vi "Intan_StreamData_parallelLoop.vi"(0 "VISA resource name":refnum<visa-resource-name>, 1 "refnum in":refnum<file>, 3 "stop":bool, 4 "Save Binary Data":bool, 5 "error in":errorcluster, 7 "byte order":T4(ring)=enum."little-endian", 8 "hdr fpath":path, 11 "DT_scale (sec)":dbl=0.01, 12 "aux file ref num":refnum<file>, 14 "save aux file":bool) -> (6 "N data scans to read (VISA)":i32=20, 10 "Nbytes VISA read":u32, 13 "VISA read iter":i32, 19 "error out":errorcluster)   [LabVIEW 2015]
doc: "Stream data to disk and user friendly display. Data is scaled and filtered prior to display.\n\nThis VI uses parallel while loop architecture: 1 loop reads from serial stream and saves raw bytes to disk; the other loop processes the data in chunk, scaling and filtering, then displays."
uses:
  zip_swcircularbuffer1_0_19b/Circular Buffer/Controls/Circular Buffer Status.ctl
  zip_swcircularbuffer1_0_19b/Circular Buffer/Controls/Circular Buffer Operations.ctl
  <vilib>/Utility/error.llb/DialogType.ctl
  zip_swcircularbuffer1_0_19b/Circular Buffer/Instance VIs/Circular Buffer(1D U16).vi
  zip_swcircularbuffer1_0_19b/Circular Buffer/Circular Buffer.lvlib
panel:
  out "setscaleresult":dbl
  out "UpdateCode":i16
  out "xmax_init":dbl
  out "offset_init":dbl
  out "increment_init":dbl
  out "xmin_init":dbl
  out "NchansChanged":bool
  out "DispLengthChanged":bool
  out "XscaleRollover":bool
  in  "Buffer Read Interval (ms)":dbl=100.0
  out "Picture":picture
  in  "Display Update interval (ms)":dbl=100.0
  in  "ChartDisplayLength (s)":dbl=5.0
  out "FS (Hz)":dbl
  out "YtxtLabelsAll":string[](array[string])
  out "error code out":i32 format="%0.0f"
  out "StopLoopsMaster":bool
  in  "Channel Select":bool
  in  "Display Chans":i32[](listbox)=[1, 4, 13, 14, 15, 16, 17, 22]
  in  "Center Traces":bool
  out "non integer read":bool
  out "N_u16s  write to buf":i32
  out "Nelements to read from buf":dbl
  out "display iter":i32
  out "% buffer full":dbl(slide) scale=0.0..100.0
  in  "Ring Buffer Size":T1={"Samples per Channel"=640000, "Channels"=0}
  out "buffer underflow":bool
  out "Buffer Status  (read)":T2
  out "buffer overflow":bool
  out "Buffer Status (write)":T2
  out "Save status":bool
  in  "Filter settings":T3={"LP Filter On/Off"=TRUE, "LP Cutoff (Hz)"=40.0, "HP Filter On/Off"=TRUE, "HP Cutoff (Hz)"=0.5, "Bandstop On/Off"=TRUE, "fl Cutoff (Hz)"=48.0, "fh Cutoff (Hz) "=52.0}
  out "N data scans to display":u16=20
  in  "offset factor":dbl=1.0
  in  "DisplayScale (uV/div)":u16(ring)=1 items=["6400", "3200", "1600", "800", "400", "200", "100", "50", "25"]
  in  "bytes per scan":i32=72
  out "timestamp_array":i32[](array[numeric])
  out "aux_cmd_array":i32[][](array[numeric])
  out "binary data (from VISA read)":u16[](array[numeric])
  in  "Nchans":i32=32
  in  "start stream (Teensy char)":string="s"
  in  "pause stream (Teensy char)":string="p"
  out "Intan Streaming Data":dbl[][](graph)
  out "Text response":string
  # "Intan-Teensy Bioelectric Module: Data Stream and Visualization"
  # "1-D data stream \nreformatted  to 2-D"
  # "Display Settings"
  # "xscale controls"
  # "Free Select"
  # "Show All"
  # "Ring Buffer Status"
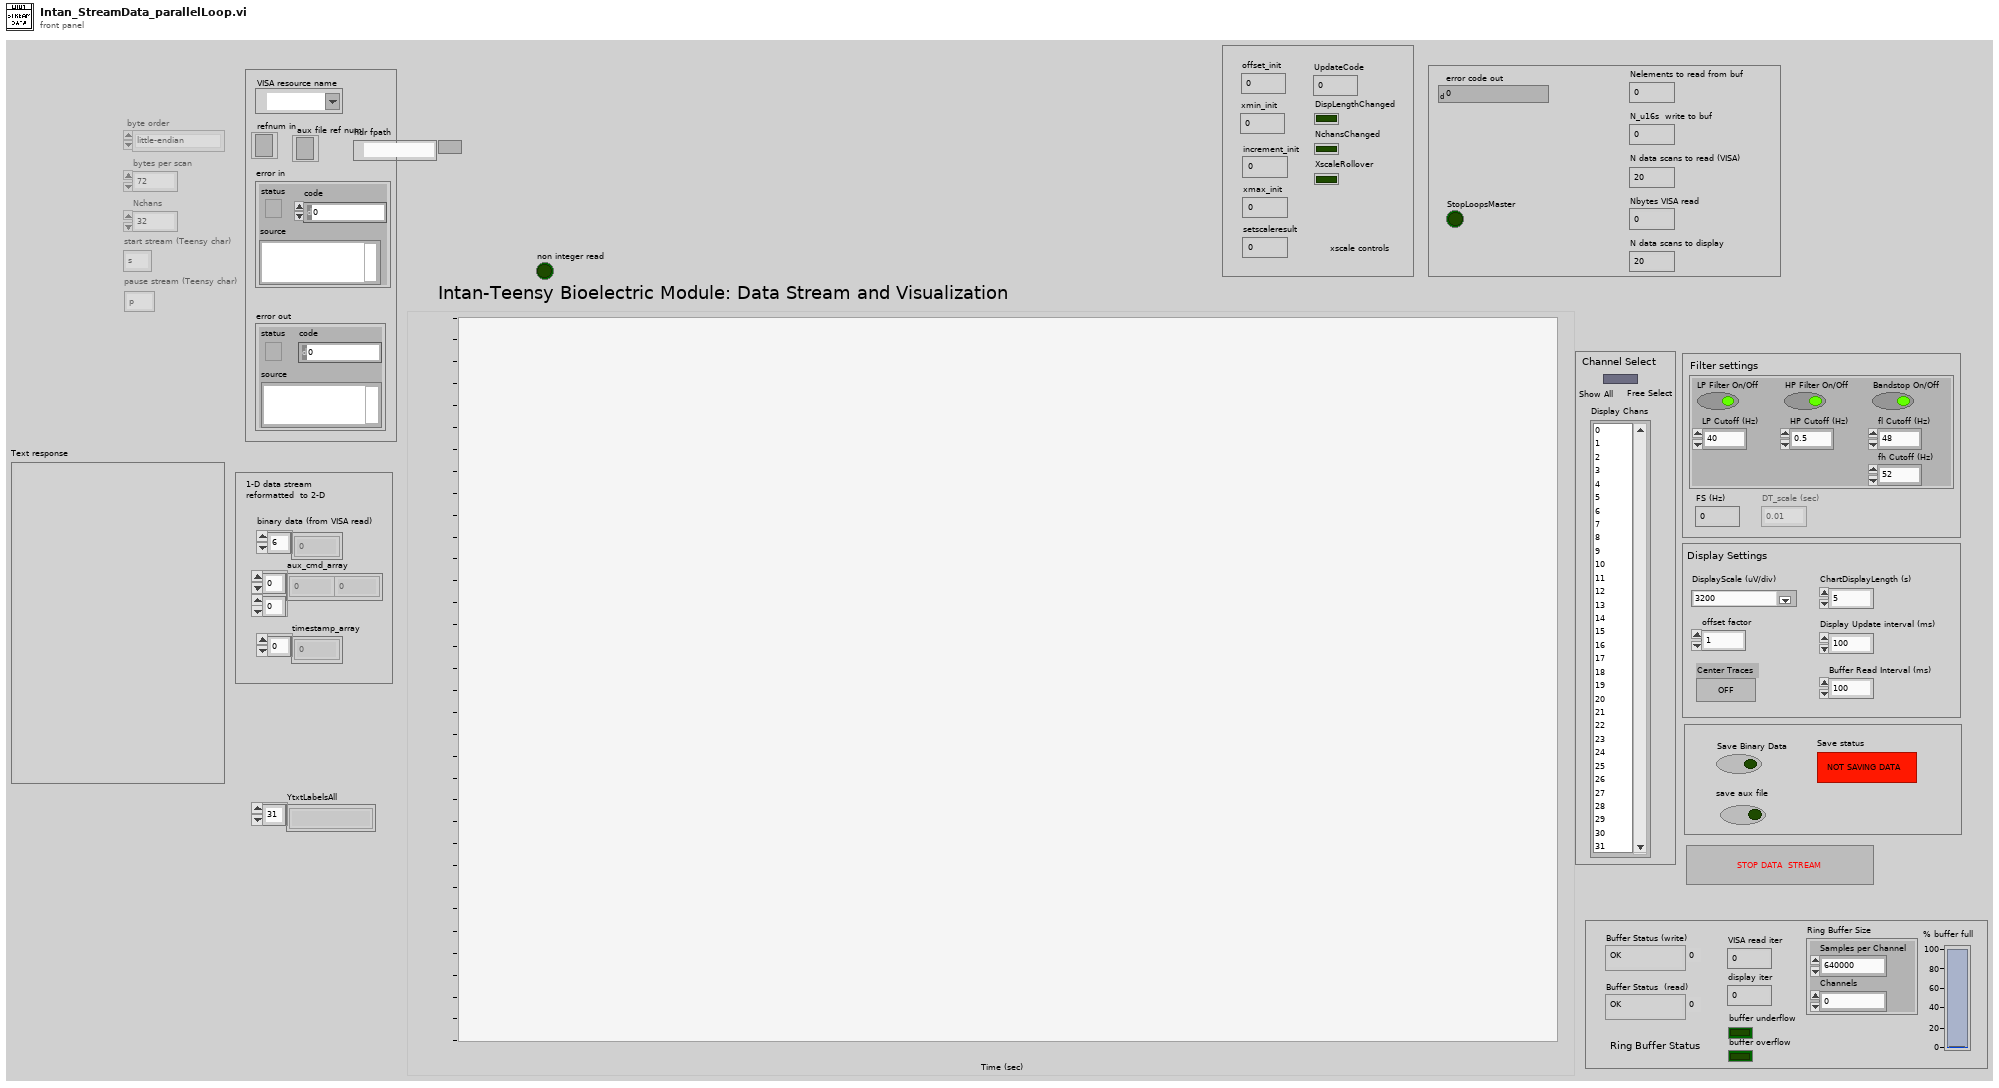
[diagram p1: front panel]
types:
  T1 = cluster{"Samples per Channel":u32, "Channels":u32}
  T2 = typedef "Circular Buffer.lvlib/Circular Buffer Status.ctl" = enum16{"OK", "Overflow", "Underflow"}
  T3 = cluster{"LP Filter On/Off":bool, "LP Cutoff (Hz)":dbl, "HP Filter On/Off":bool, "HP Cutoff (Hz)":dbl, "Bandstop On/Off":bool, "fl Cutoff (Hz)":dbl, "fh Cutoff (Hz) ":dbl}
  T4 = enum16{"big-endian, network order", "native, host order", "little-endian"}
  T5 = typedef "Circular Buffer.lvlib/Circular Buffer Operations.ctl" = enum16{"Initialize", "Get Backlog", "Write", "Read (continuous)", "Read (most recent)"}
  T6 = typedef "LVRectTypeDef.ctl" = cluster{"Left":i16, "Top":i16, "Right":i16, "Bottom":i16}
  T7 = typedef "DialogType.ctl" = u16
  T8 = cluster{"XScale.Minimum":dbl, "XScale.Maximum":dbl, "XScale.Increment":dbl, "Nchannels":i32}
  T9 = cluster{"Maximum":dbl, dbl, dbl, dbl, dbl, dbl, "YscleMark":dbl, "Increment":dbl}
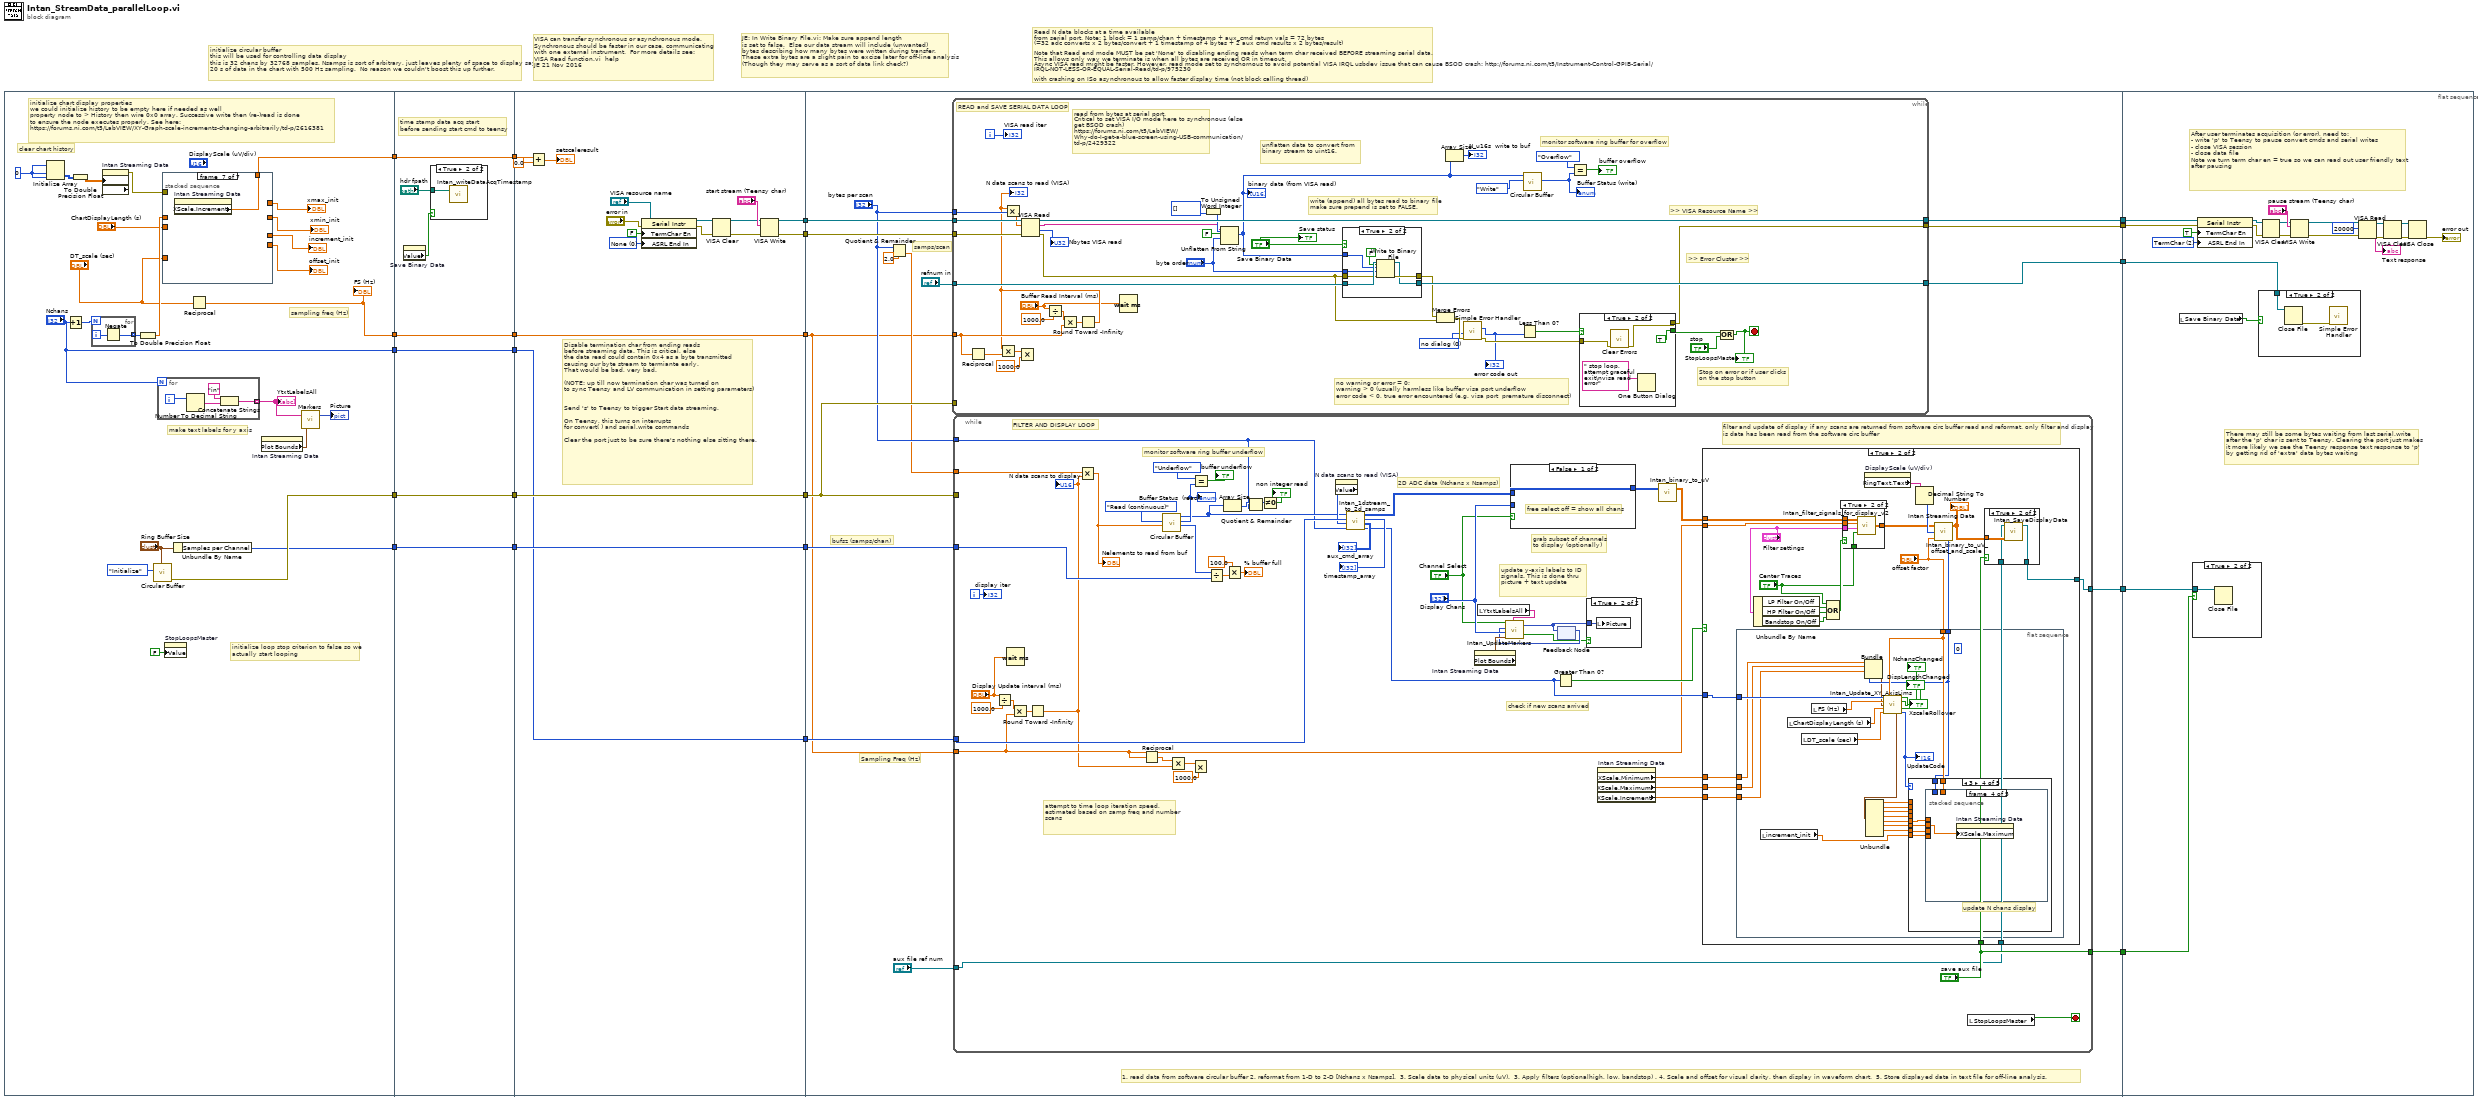
[diagram p0: block diagram]
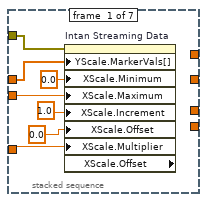
[diagram p2: hidden frame]
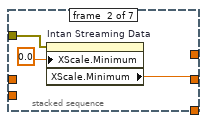
[diagram p3: hidden frame]
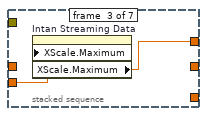
[diagram p4: hidden frame]
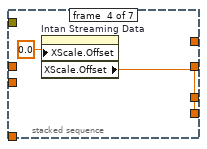
[diagram p5: hidden frame]
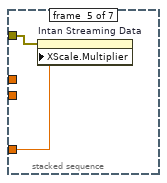
[diagram p6: hidden frame]
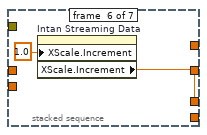
[diagram p7: hidden frame]
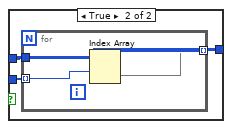
[diagram p10: hidden frame]
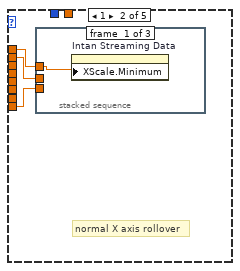
[diagram p13: hidden frame]
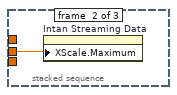
[diagram p14: hidden frame]
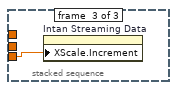
[diagram p15: hidden frame]
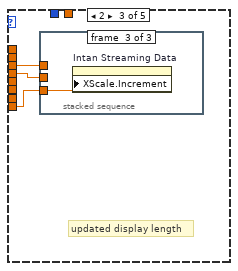
[diagram p16: hidden frame]
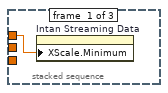
[diagram p17: hidden frame]
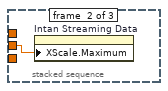
[diagram p18: hidden frame]
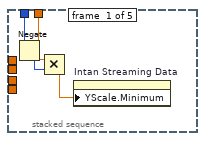
[diagram p19: hidden frame]
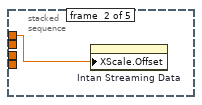
[diagram p20: hidden frame]
diagram:
  # "Read N data blocks at a time available\nfrom serial port. Note: 1 block = 1 samp/chan + timestamp + aux_cmd return vals = 72 bytes \n(=32 adc converts x 2 bytes/convert + 1 timestamp of 4 bytes + 2 aux cmd results x 2 bytes/result) \n\nNote that Read end mode MUST be set 'None' to disabling ending reads when term char received BEFORE streaming serial data.  \nThis allows only way we terminate is when all bytes are received OR in timeout.  \nAsync VISA read might be faster. However, read mode set to synchornous to avoid potential VISA IRQL usbdev issue that can cause BSOD crash: http://forums.ni.com/t5/Instrument-Control-GPIB-Serial/IRQL-NOT-LESS-OR-EQUAL-Serial-Read/td-p/975230\n\nwith crashing on ISo asynchronous to allow faster display time (not block calling thread)"
  # "initialize circular buffer\nthis will be used for controlling data display\nthis is 32 chans by 32768 samples. Nsamps is sort of arbitrary, just leaves plenty of space to display say\n20 s of data in the chart with 500 Hz sampling.  No reason we couldn't boost this up further."
  # "JE: In Write Binary File.vi: Make sure append length \nis set to false.  Else our data stream will include (unwanted)\nbytes describing how many bytes were written during transfer.\nThese extra bytes are a slight pain to excise later for off-line analysis\n(Though they may serve as a sort of data link check?)"
  # "VISA can transfer synchronous or asynchronous mode.\nSynchronous should be faster in our case, communicating\nwith one external instrument.  For more details see: \nVISA Read function.vi  help \nJE 21 Nov 2016"
  n1 = flat-sequence {
    tunnel: [w42] -> w10
    tunnel: [w40] -> w8
    tunnel: ["Nchans"] -> w6
    tunnel: [w34] -> w4
    tunnel: [w22] -> w2
    tunnel: w10 -> [w77]
    tunnel: [w77] -> w9
    tunnel: w8 -> [w76]
    tunnel: [w76] -> w7
    tunnel: w6 -> [w75]
    tunnel: [w75] -> w5
    tunnel: w4 -> [w74]
    tunnel: [w74] -> w3
    tunnel: w2 -> [w73]
    tunnel: [w73] -> w1
    tunnel: [w86] -> w19
    tunnel: [w87] -> w18
    tunnel: [w85] -> w17
    tunnel: w9 -> [w85]
    tunnel: [w84] -> w16
    tunnel: w7 -> [w84]
    tunnel: w5 -> [w83]
    tunnel: [w83] -> w15
    tunnel: [w82] -> w14
    tunnel: w3 -> [w82]
    tunnel: w1 -> [w81]
    tunnel: [w108] -> w21
    tunnel: [w111] -> w20
    tunnel: w19 -> [w109]
    tunnel: w18 -> [w110]
    tunnel: w17 -> [w107]
    tunnel: w16 -> [w105]
    tunnel: w15 -> [w104]
    tunnel: w14 -> [w101]
    tunnel: [w100] -> w13
    tunnel: [w98] -> w12
    tunnel: [w97] -> w11
    tunnel: w21 -> [w331]
    tunnel: w20 -> [w344]
    tunnel: w13 -> [w326]
    tunnel: w12 -> [w325]
    tunnel: w11 -> [w324]
    frame #0 {
      w33 = 0 ("Dimension Size")
      # "clear chart history"
      # "initialize loop stop criterion to false so we\nactually start looping"
      # "make text labels for y axis"
      # "sampling freq (Hz)"
      # "initialize chart display properties\nwe could initialize history to be empty here if needed as well\nproperty node to > History then wire 0x0 array. Successive write then (re-)read is done\nto ensure the node executes properly. See here:\nhttps://forums.ni.com/t5/LabVIEW/XY-Graph-scale-increments-changing-arbitrarily/td-p/2616381"
      n2 = Initialize Array(w33, w33, w33) -> (w32:i32[][])
      n3 = Increment(x="Nchans") -> (x+1=w44:i32)
      n4 = To Double Precision Float(number=w32) -> (double precision float=w30:dbl[][])
      n5 = for {
        N: w44 -> [_]
        tunnel: [w69] -> w45 mode=indexing
        i -> [w70]
        n6 = Negate(x=w70) -> (-x=w69:i32)
      }
      n7 = property on="Intan Streaming Data" class="WFChart (strict)" props=["History Data", "History Data"]("History Data"=w30) -> (error out=w29:errorcluster)  [unwired: 2 in, 2 out]
      n8 = To Double Precision Float(number=w45) -> (double precision float=w31:dbl[])
      n9 = call-poly "Circular Buffer.vi"("Buffer Size"="Ring Buffer Size", "Operation"=Circular_Buffer_Operations."Initialize") -> ("error out"=w42:errorcluster)  [unwired: 6 in, 3 out]
      n10 = for {
        N: "Nchans" -> [_]
        tunnel: [w66] -> w37 mode=indexing
        i -> [w65]
        n11 = Number To Decimal String(number=w65) -> (decimal integer string=w68:string)  [unwired: 1 in]
        n12 = Concatenate Strings("in" ("string"), w68) -> (w66:string)
      }
      "YtxtLabelsAll" <- w37
      n13 = stacked-sequence {
        tunnel: w31 -> [w52 _ _ _ _ _ _]
        tunnel: w29 -> [w51 w54 _ _ w60 _ _]
        tunnel: "ChartDisplayLength (s)" -> [w49 _ w57 _ _ _ _]
        tunnel: "DT_scale (sec)" -> [w48 _ _ _ w61 _ _]
        tunnel: [_ _ w56 _ _ _ _] -> w23
        tunnel: [_ w55 _ _ _ _ _] -> w26
        tunnel: [_ _ _ _ _ w62 _] -> w25
        tunnel: [_ _ _ w58 _ _ _] -> w24
        tunnel: [_ _ _ _ _ _ w64] -> w22
        frame #0 {
          n14 = property on="Intan Streaming Data" class="WFChart (strict)" props=["YScale", "MarkerVals[]", "XScale", "Minimum", "XScale", "Maximum", "XScale", "Increment", "XScale", "Offset", "XScale", "Multiplier", "XScale", "Offset"](error in=w51, "YScale.MarkerVals[]"=w52, "XScale.Minimum"=0.0 ("X Scale.Range:Minimum"), "XScale.Maximum"=w49, "XScale.Increment"=1.0 ("X Scale.Range:Minimum"), "XScale.Offset"=0.0 ("X Scale.Range:Minimum"), "XScale.Multiplier"=w48) -> ()  [unwired: 1 in, 3 out]
        }
        frame #1 {
          n15 = property on="Intan Streaming Data" class="WFChart (strict)"(error in=w54, "XScale.Minimum"=0.0 ("X Scale.Range:Minimum")) -> ("XScale.Minimum"=w55:dbl)  [unwired: 1 in, 2 out]
        }
        frame #2 {
          n16 = property on="Intan Streaming Data" class="WFChart (strict)"("XScale.Maximum"=w57) -> ("XScale.Maximum"=w56:dbl)  [unwired: 2 in, 2 out]
        }
        frame #3 {
          n17 = property on="Intan Streaming Data" class="WFChart (strict)"("XScale.Offset"=0.0 ("X Scale.Offset and Multiplier:Offset")) -> ("XScale.Offset"=w58:dbl)  [unwired: 2 in, 2 out]
        }
        frame #4 {
          n18 = property on="Intan Streaming Data" class="WFChart (strict)"(error in=w60, "XScale.Multiplier"=w61) -> ()  [unwired: 1 in, 2 out]
        }
        frame #5 {
          n19 = property on="Intan Streaming Data" class="WFChart (strict)"("XScale.Increment"=1.0 ("X Scale.Range:Increment")) -> ("XScale.Increment"=w62:dbl)  [unwired: 2 in, 2 out]
        }
        frame #6 {
          n20 = property on="Intan Streaming Data" class="WFChart (strict)"() -> ("XScale.Increment"=w64:dbl)  [unwired: 2 in, 2 out]
        }
      }
      "xmin_init" <- w26
      "increment_init" <- w25
      "offset_init" <- w24
      "xmax_init" <- w23
      n21 = property on="StopLoopsMaster" class="Bool (strict)"("Value"=FALSE ("StopLoopsMaster")) -> ()  [unwired: 2 in, 2 out]
      n22 = Unbundle By Name("Ring Buffer Size") -> ("Samples per Channel"=w40:u32)
      n23 = Reciprocal(x="DT_scale (sec)") -> (1/x=w34:dbl)
      "FS (Hz)" <- w34
      n24 = property on="Intan Streaming Data" class="WFChart (strict)"() -> ("Plot Bounds"=w35:T6)  [unwired: 2 in, 2 out]
      n25 = call "Markers.vi"("plot bounds"=w35, "Array"=w37) -> ("Picture"=→"Picture":picture)  [unwired: 1 out]
    }
    frame #1 {
      # "time stamp data acq start\nbefore sending start cmd to teensy"
      n26 = property on="Save Binary Data" class="Bool (strict)"() -> ("Value"=w72:bool)  [unwired: 2 in, 2 out]
      n27 = case shown="True" w72 {
        tunnel: "hdr fpath" -> [_ w78]
        frame False {
        }
        frame True {
          n28 = call "Intan_writeDataAcqTimestamp.vi"("hdr fpath"=w78) -> ()  [unwired: 2 in, 1 out]
        }
      }
    }
    frame #2 {
      w92 = u16 0 items=["None", "Last Bit", "TermChar"] ("Serial Settings:End Mode for Reads")
      # "Disable termination char from ending reads\nbefore streaming data. This is critical, else\nthe data read could contain 0x4 as a byte transmitted\ncausing our byte stream to termiante early.\nThat would be bad, very bad.\n\n(NOTE: up till now termination char was turned on\nto sync Teensy and LV communication in setting parameters)\n\n\nSend 's' to Teensy to trigger Start data streaming.  \n\nOn Teensy, this turns on interrupts\nfor convert( ) and serial.write commands\n\nClear the port just to be sure there's nothing else sitting there."
      n29 = Add(x=w81, y=0.0) -> (x+y=→"setscaleresult":dbl)
      n30 = property class="Serial Instr"(reference="VISA resource name", error in="error in", "TermChar En"=FALSE ("Message Based Settings:Termination Character Enable"), "ASRL End In"=w92) -> (reference out=w91:refnum<visa-resource-name>, error out=w90:errorcluster)
      n31 = VISA Clear(VISA resource name=w91, error in (no error)=w90) -> (VISA resource name out=w89:refnum<visa-resource-name>, error out=w88:errorcluster)
      n32 = VISA Write(VISA resource name=w89, write buffer="start stream (Teensy char)", error in (no error)=w88) -> (VISA resource name out=w87:refnum<visa-resource-name>, error out=w86:errorcluster)  [unwired: 1 out]
    }
    frame #3 {
      # "1. read data from software circular buffer 2. reformat from 1-D to 2-D [Nchans x Nsamps].  3. Scale data to physical units (uV).  3. Apply filters (optionalhigh, low, bandstop) . 4. Scale and offset for visual clarity, then display in waveform chart.  5. Store displayed data in text file for off-line analysis."
      # "Sampling Freq (Hz)"
      # "bufsz (samps/chan)"
      # "samps/scan"
      n33 = Quotient & Remainder(x="bytes per scan", y=2.0) -> (floor(x/y)=w102:dbl)  [unwired: 1 out]
      n34 = while {
        tunnel: [w307] -> w108
        tunnel: [w305] -> w111
        tunnel: w109 -> [w301]
        tunnel: "refnum in" -> [w304]
        tunnel: w110 -> [w302]
        tunnel: w107 -> [_]
        tunnel: "bytes per scan" -> [w286]
        tunnel: w101 -> [w269]
        tunnel: [w273] -> w98
        i -> [w303]
        stop <- w306 stop-if-true
        w279 = T7 0 items=["no dialog", "OK message", "continue or stop message", "OK message + warnings", "continue/stop + warnings"] ("type of dialog (OK msg:1)")
        # "no warning or error = 0;\nwarning > 0 (usually harmless like buffer visa port underflow\nerror code < 0, true error encountered (e.g. visa port  premature disconnect)"
        # "READ and SAVE SERIAL DATA LOOP"
        # "monitor software ring buffer for overflow"
        # "write (append) all bytes read to binary file\nmake sure prepend is set to FALSE."
        # "unflatten data to convert from binary stream to uint16."
        # "Stop on error or if user clicks \non the stop button"
        # ">> Error Cluster >>"
        # ">> VISA Resource Name >>"
        # "read from bytes at serial port.\nCritical to set VISA I/O mode here to synchronous (else get BSOD crash)\nhttps://forums.ni.com/t5/LabVIEW/Why-do-I-get-a-blue-screen-using-USB-communication/td-p/2429322"
        n35 = Reciprocal(x=w269) -> (1/x=w283:dbl)
        n36 = Divide(x="Buffer Read Interval (ms)", y=1000.0) -> (x/y=w271:dbl)
        n37 = Multiply(x=w271, y=w269) -> (x*y=w272:dbl)
        n38 = Round Toward -Infinity(1:w272) -> (0:w268:dbl)
        "N data scans to read (VISA)" <- w268
        n39 = Multiply(x=w268, y=w283) -> (x*y=w285:dbl)
        n40 = Multiply(x=w268, y=w286) -> (x*y=w287:dbl)
        n41 = Multiply(x=w285, y=1000.0) -> ()  [unwired: 1 out]
        n42 = VISA Read(VISA resource name=w302, byte count=w287, error in (no error)=w301) -> (VISA resource name out=w307:refnum<visa-resource-name>, read buffer=w295:string, return count=→"Nbytes VISA read":u32, error out=w281:errorcluster)
        n43 = Wait (ms)(milliseconds to wait="Buffer Read Interval (ms)") -> ()  [unwired: 1 out]
        n44 = To Unsigned Word Integer(number=i16[] []) -> (unsigned 16bit integer=w297:u16[])
        n45 = Unflatten From String(type=w297, binary string=w295, data includes array or string size? (T)=FALSE, byte order (0:big-endian, network order)="byte order") -> (value=w289:u16[])  [unwired: 1 in, 2 out]
        "binary data (from VISA read)" <- w289
        n46 = case shown="True" "Save Binary Data" {
          tunnel: [w315 w322] -> w282
          tunnel: [w314 w321] -> w305
          tunnel: w304 -> [w314 w320]
          tunnel: w281 -> [w315 w319]
          tunnel: "byte order" -> [_ w317]
          tunnel: w289 -> [_ w316]
          frame False {
          }
          frame True {
            n47 = Write to Binary File(file (use dialog)=w320, data=w316, error in=w319, 5:FALSE ("prepend array or string size? (T)"), 9:w317) -> (refnum out=w321:refnum<file>, error out=w322:errorcluster)  [unwired: 1 in, 1 out]
          }
        }
        n48 = Merge Errors(w282, w281) -> (w280:errorcluster)
        n49 = Array Size(array=w289) -> (size(s)=→"N_u16s  write to buf":i32)
        n50 = call <vilib>:"Simple Error Handler.vi"("type of dialog (OK msg:1)"=w279, "error in (no error)"=w280) -> ("code out"=w276:i32, "error out"=w277:errorcluster)  [unwired: 3 in, 3 out]
        "error code out" <- w276
        n51 = Less Than 0?(x=w276) -> (x < 0?=w274:bool)
        n52 = call-poly "Circular Buffer.vi"("Operation"=Circular_Buffer_Operations."Write", "Data In"=w289) -> ("Buffer Status"=w291:T2)  [unwired: 6 in, 3 out]
        "Buffer Status (write)" <- w291
        n53 = Equal?(x=Circular_Buffer_Status."Overflow" ("y"), y=w291) -> (x = y?=→"buffer overflow":bool)
        n54 = case shown="True" w274 {
          tunnel: w277 -> [w308 w312]
          tunnel: [FALSE TRUE] -> w275
          tunnel: [w308 w310] -> w273
          frame False {
          }
          frame True {
            n55 = call <vilib>:"Clear Errors.vi"("error in (no error)"=w312) -> ("error out"=w310:errorcluster)  [unwired: 5 in, 1 out]
            n56 = One Button Dialog(message=" stop loop, attempt graceful exit\nvisa read error") -> ()  [unwired: 1 in, 1 out]
          }
        }
        n57 = Compound Arithmetic op=OR(w275, "stop") -> (w306:bool)
        "StopLoopsMaster" <- w306
        "VISA read iter" <- w303
        "Save status" <- "Save Binary Data"
      }
      n58 = while {
        tunnel: w107 -> [_]
        tunnel: w105 -> [w156]
        tunnel: w104 -> [w152]
        tunnel: "bytes per scan" -> [w142]
        tunnel: w101 -> [w121]
        tunnel: w102 -> [w148]
        tunnel: [w127] -> w100
        tunnel: "aux file ref num" -> [w126]
        tunnel: ["save aux file"] -> w97
        i -> [w149]
        stop <- w124 stop-if-true
        # "2D ADC data (Nchans x Nsamps)"
        # "check if new scans arrived"
        # "grab subset of channels\nto display (optionally)"
        # "update y-axis labels to ID signals. This is done thru picture + text update"
        # "FILTER AND DISPLAY LOOP"
        # "attempt to time loop iteration speed,\nestimated based on samp freq and number scans"
        # "filter and update of display if any scans are returned from software circ buffer read and reformat. only filter and display is data has been read from the software circ buffer"
        # "monitor software ring buffer underflow"
        n59 = Divide(x="Display Update interval (ms)", y=1000.0) -> (x/y=w118:dbl)
        n60 = Wait (ms)(milliseconds to wait="Display Update interval (ms)") -> ()  [unwired: 1 out]
        n61 = Multiply(x=w118, y=w121) -> (x*y=w120:dbl)
        n62 = Round Toward -Infinity(1:w120) -> (0:w119:dbl)
        "N data scans to display" <- w119
        n63 = Multiply(x=w148, y=w119) -> (x*y=w147:dbl)
        "Nelements to read from buf" <- w147
        n64 = Reciprocal(x=w121) -> (1/x=w139:dbl)
        n65 = call-poly "Circular Buffer.vi"("Read Size"=w147, "Operation"=Circular_Buffer_Operations."Read (continuous)") -> ("Elements Remaining"=w157:i32, "Buffer Status"=w159:T2, "Data Out"=w144:u16[])  [unwired: 6 in, 1 out]
        "Buffer Status  (read)" <- w159
        n66 = Multiply(x=w139, y=w119) -> (x*y=w138:dbl)
        n67 = Multiply(x=w138, y=1000.0) -> ()  [unwired: 1 out]
        n68 = Equal?(x=Circular_Buffer_Status."Underflow" ("y"), y=w159) -> (x = y?=→"buffer underflow":bool)
        n69 = Divide(x=w157, y=w156) -> (x/y=w155:dbl)
        n70 = Array Size(array=w144) -> (size(s)=w143:i32)
        n71 = Multiply(x=100.0, y=w155) -> (x*y=→"% buffer full":dbl)
        n72 = Quotient & Remainder(x=w143, y=w142) -> (x-y*floor(x/y)=w141:i32)  [unwired: 1 out]
        n73 = Not Equal To 0?(x=w141) -> (x != 0?=→"non integer read":bool)
        n74 = property on="N data scans to read (VISA)" class="DigNum (strict)"() -> ("Value"=w146:i32)  [unwired: 2 in, 2 out]
        n75 = call "Intan_1dstream_to_2d_samps.vi"("bytes per scan"=w142, "N data scans to read"=w146, "Nchans"=w152, "1-D  data in"=w144) -> ("Nscans read"=w125:i32, "aux_cmd_array"=→"aux_cmd_array":i32[][], "timestamp_array"=→"timestamp_array":i32[], "2d ADCdata_array out"=w136:u16[][])  [unwired: 2 in, 2 out]
        n76 = property on="Intan Streaming Data" class="WFChart (strict)"() -> ("Plot Bounds"=w133:T6)  [unwired: 2 in, 2 out]
        n77 = local read "YtxtLabelsAll"() -> (w122:string[])
        n78 = case shown="False" "Channel Select" {
          tunnel: w136 -> [w163 w166]
          tunnel: [w163 w165] -> w123
          tunnel: "Display Chans" -> [_ w164]
          frame False {
            # "free select off = show all chans"
          }
          frame True {
            n79 = for {
              tunnel: w166 -> [w169]
              tunnel: w164 -> [w167] mode=indexing
              tunnel: [w168] -> w165 mode=indexing
              n80 = Index Array(array=w169, index (row)=w167) -> (element=w168:u16[])  [unwired: 1 in]
            }
          }
        }
        n81 = Greater Than 0?(x=w125) -> (x > 0?=w145:bool)
        n82 = feedback #1() -> (w132:picture)  [unwired: 1 in]
        n83 = call "Intan_UpdateMarkers.vi"("Free Select Chans"="Channel Select", "Picture In"=w132, "Display Chans"="Display Chans", "plot bounds"=w133, "YtxtLabelsAll"=w122) -> ("Picture Out"=w129:picture, "update labels"=w130:bool)
        n84 = feedback-in #1(w129) -> ()
        n85 = case shown="True" w130 {
          tunnel: w129 -> [_ w162]
          frame False {
          }
          frame True {
            n86 = local write "Picture"(w162) -> ()
          }
        }
        n87 = property on="Intan Streaming Data" class="WFChart (strict)"() -> ("XScale.Minimum"=w115:dbl, "XScale.Maximum"=w114:dbl, "XScale.Increment"=w113:dbl)  [unwired: 2 in, 2 out]
        n88 = call "Intan_binary_to_uV.vi"("2d ADC binary data"=w123) -> ("Scaled Data (uV)"=w135:dbl[][])  [unwired: 2 in]
        n89 = case shown="True" w145 {
          tunnel: w121 -> [_ w190]
          tunnel: w135 -> [_ w188]
          tunnel: [w170 w181] -> w127
          tunnel: "save aux file" -> [_ w180]
          tunnel: w126 -> [w170 w179]
          tunnel: w125 -> [_ w177]
          tunnel: w115 -> [_ w173]
          tunnel: w114 -> [_ w172]
          tunnel: w113 -> [_ w171]
          frame False {
          }
          frame True {
            n90 = flat-sequence {
              tunnel: w177 -> [w212]
              tunnel: "offset factor" -> [w199]
              tunnel: w174 -> [w196]
              tunnel: w173 -> [w194]
              tunnel: w172 -> [w193]
              tunnel: w171 -> [w192]
              frame #0 {
                (unwired) 0 ("index")
                n91 = local read "increment_init"() -> (w198:dbl)
                n92 = local read "ChartDisplayLength (s)"() -> (w210:dbl)
                n93 = local read "DT_scale (sec)"() -> (w209:dbl)
                n94 = local read "FS (Hz)"() -> (w211:dbl)
                n95 = Bundle("XScale.Minimum"=w194, "XScale.Maximum"=w193, "XScale.Increment"=w192, "Nchannels"=w196) -> (w195:T8)  [unwired: 1 in]
                n96 = call "Intan_Update_XY_AxisLims.vi"("NscansRead"=w212, "offset factor"=w199, "FS (Hz)"=w211, "XscaleClusterCurrent"=w195, "DisplayLength(s)"=w210, "DT_scale (s)"=w209) -> ("XscaleRollover"=→"XscaleRollover":bool, "DispLengthChanged"=→"DispLengthChanged":bool, "NchansChanged"=→"NchansChanged":bool, "XYlims Update Cluster"=w207:T9, "UpdateCode"=w208:i16)  [unwired: 4 in, 1 out]
                "UpdateCode" <- w208
                n97 = Unbundle(w207) -> ("Maximum"=w204:dbl, w203:dbl, w201:dbl, w200:dbl, w206:dbl, w205:dbl, "YscleMark"=w202:dbl)  [unwired: 1 out]
                n98 = case shown="3" w208 {
                  tunnel: w196 -> [_ _ _ w232 w243]
                  tunnel: w206 -> [_ _ _ w227 _]
                  tunnel: w205 -> [_ _ _ w231 _]
                  tunnel: w204 -> [_ w217 _ _ w246]
                  tunnel: w203 -> [_ w216 _ _ w245]
                  tunnel: w202 -> [_ _ _ w230 w244]
                  tunnel: w201 -> [_ _ w222 _ _]
                  tunnel: w200 -> [_ _ w223 _ _]
                  tunnel: w199 -> [_ _ _ w229 w242]
                  tunnel: w198 -> [_ w215 w221 w228 w241]
                  frame 0, Default {
                    # "nothing to update"
                  }
                  frame 1 {
                    # "normal X axis rollover"
                    n99 = stacked-sequence {
                      tunnel: w217 -> [w218 _ _]
                      tunnel: w216 -> [_ w219 _]
                      tunnel: w215 -> [_ _ w220]
                      frame #0 {
                        n100 = property on="Intan Streaming Data" class="WFChart (strict)"("XScale.Minimum"=w218) -> ()  [unwired: 2 in, 2 out]
                      }
                      frame #1 {
                        n101 = property on="Intan Streaming Data" class="WFChart (strict)"("XScale.Maximum"=w219) -> ()  [unwired: 2 in, 2 out]
                      }
                      frame #2 {
                        n102 = property on="Intan Streaming Data" class="WFChart (strict)"("XScale.Increment"=w220) -> ()  [unwired: 2 in, 2 out]
                      }
                    }
                  }
                  frame 2 {
                    # "updated display length"
                    n103 = stacked-sequence {
                      tunnel: w221 -> [_ _ w226]
                      tunnel: w223 -> [_ w225 _]
                      tunnel: w222 -> [w224 _ _]
                      frame #0 {
                        n104 = property on="Intan Streaming Data" class="WFChart (strict)"("XScale.Minimum"=w224) -> ()  [unwired: 2 in, 2 out]
                      }
                      frame #1 {
                        n105 = property on="Intan Streaming Data" class="WFChart (strict)"("XScale.Maximum"=w225) -> ()  [unwired: 2 in, 2 out]
                      }
                      frame #2 {
                        n106 = property on="Intan Streaming Data" class="WFChart (strict)"("XScale.Increment"=w226) -> ()  [unwired: 2 in, 2 out]
                      }
                    }
                  }
                  frame 3 {
                    # "update N chans display"
                    n107 = stacked-sequence {
                      tunnel: w232 -> [w236 _ _ _ _]
                      tunnel: w228 -> [_ _ _ _ w240]
                      tunnel: w231 -> [_ _ _ w239 _]
                      tunnel: w230 -> [_ _ _ _ _]
                      tunnel: w229 -> [w234 _ _ _ _]
                      tunnel: w227 -> [_ w237 w238 _ _]
                      frame #0 {
                        n108 = Negate(x=w236) -> (-x=w235:i32)
                        n109 = Multiply(x=w234, y=w235) -> (x*y=w233:dbl)
                        n110 = property on="Intan Streaming Data" class="WFChart (strict)"("YScale.Minimum"=w233) -> ()  [unwired: 2 in, 2 out]
                      }
                      frame #1 {
                        n111 = property on="Intan Streaming Data" class="WFChart (strict)"("XScale.Offset"=w237) -> ()  [unwired: 2 in, 2 out]
                      }
                      frame #2 {
                        n112 = property on="Intan Streaming Data" class="WFChart (strict)"("XScale.Minimum"=w238) -> ()  [unwired: 2 in, 2 out]
                      }
                      frame #3 {
                        n113 = property on="Intan Streaming Data" class="WFChart (strict)"("XScale.Maximum"=w239) -> ()  [unwired: 2 in, 2 out]
                      }
                      frame #4 {
                        n114 = property on="Intan Streaming Data" class="WFChart (strict)"("XScale.Increment"=w240) -> ()  [unwired: 2 in, 2 out]
                      }
                    }
                  }
                  frame 4 {
                    # "updated offset factor"
                    n115 = stacked-sequence {
                      seq-local: [w247 _ _] -> [_ w251 _]
                      tunnel: w246 -> [_ _ _]
                      tunnel: w245 -> [_ _ _]
                      tunnel: w244 -> [_ _ _]
                      tunnel: w243 -> [w250 _ _]
                      tunnel: w242 -> [w248 _ _]
                      tunnel: w241 -> [_ _ w256]
                      frame #0 {
                        n116 = Negate(x=w250) -> (-x=w249:i32)
                        n117 = Multiply(x=w248, y=w249) -> (x*y=w247:dbl)
                        n118 = property on="Intan Streaming Data" class="WFChart (strict)"("YScale.Minimum"=w247) -> ()  [unwired: 2 in, 2 out]
                      }
                      frame #1 {
                        n119 = for {
                          N: w251 -> [_]
                          tunnel: [w254] -> w253 mode=indexing
                          i -> [w255]
                          n120 = Negate(x=w255) -> (-x=w254:i32)
                        }
                        n121 = To Double Precision Float(number=w253) -> (double precision float=w252:dbl[])
                        n122 = property on="Intan Streaming Data" class="WFChart (strict)" props=["YScale", "MarkerVals[]", "YScale", "MarkerVals[]"]("YScale.MarkerVals[]"=w252) -> ()  [unwired: 2 in, 3 out]
                      }
                      frame #2 {
                        n123 = property on="Intan Streaming Data" class="WFChart (strict)"("XScale.Increment"=w256) -> ()  [unwired: 2 in, 2 out]
                      }
                    }
                  }
                }
              }
            }
            n124 = Unbundle By Name("Filter settings") -> ("LP Filter On/Off"=w186:bool, "HP Filter On/Off"=w185:bool, "Bandstop On/Off"=w183:bool)
            n125 = Compound Arithmetic op=OR("Center Traces", w186, w185, w183) -> (w184:bool)
            n126 = case shown="True" w184 {
              tunnel: w190 -> [_ w266]
              tunnel: w188 -> [w261 w265]
              tunnel: [w261 w264] -> w178
              tunnel: "Filter settings" -> [_ w263]
              tunnel: "Center Traces" -> [_ w262]
              frame False {
              }
              frame True {
                n127 = call "Intan_filter_signals_for_display_v2.vi"("Center Traces"=w262, "input filter cluster"=w263, "Sample Rate (Hz)"=w266, "Nchan Array In [Nchans x Nsamps]"=w265) -> ("Display Signals Out [Nchans x Nsamps]"=w264:dbl[][])
              }
            }
            n128 = property on="DisplayScale (uV/div)" class="Ring (strict)"() -> ("RingText.Text"=w189:string)  [unwired: 2 in, 2 out]
            n129 = Decimal String To Number(string=w189) -> (number=w191:i32)  [unwired: 2 in, 1 out]
            n130 = call "Intan_binary_to_uV_offset_and_scale.vi"("offset spacing factor"="offset factor", "Yscale (uv/div)"=w191, "ScaledData [Nchans x Nsamps]"=w178) -> ("Nchannels"=w174:i32, "Data4Display"=w176:dbl[][])  [unwired: 1 in]
            "Intan Streaming Data" <- w176
            n131 = case shown="True" w180 {
              tunnel: w176 -> [_ w260]
              tunnel: [w257 w259] -> w181
              tunnel: w179 -> [w257 w258]
              frame False {
              }
              frame True {
                n132 = call "Intan_SaveDisplayData.vi"("2d ADCdata_array out"=w260, "aux file ref num"=w258) -> ("refnum out"=w259:refnum<file>)  [unwired: 3 in]
              }
            }
          }
        }
        n133 = local read "StopLoopsMaster"() -> (w124:bool)
        "display iter" <- w149
      }
    }
    frame #4 {
      w336 = u16 2 items=["None", "Last Bit", "TermChar"] ("Serial Settings:End Mode for Reads")
      # "There may still be some bytes waiting from last serial.write\nafter the 'p' char is sent to Teensy. Clearing the port just makes\nit more likely we see the Teensy response text response to 'p' \nby getting rid of 'extra' data bytes waiting"
      # "After user terminates acquisition (or error), need to:\n- write 'p' to Teensy to pause convert cmds and serial writes\n- close VISA session\n- close data file\nNote we turn term char en = true so we can read out user friendly text \nafter pausing"
      n134 = local read "Save Binary Data"() -> (w323:bool)
      n135 = case shown="True" w324 {
        tunnel: w326 -> [_ w347]
        frame False {
        }
        frame True {
          n136 = Close File(refnum=w347) -> ()  [unwired: 1 in, 2 out]
        }
      }
      n137 = property class="Serial Instr"(reference=w331, error in=w325, "TermChar En"=TRUE ("Message Based Settings:Termination Character Enable"), "ASRL End In"=w336) -> (reference out=w330:refnum<visa-resource-name>, error out=w329:errorcluster)
      n138 = case shown="True" w323 {
        tunnel: w344 -> [_ w345]
        frame False {
        }
        frame True {
          n139 = Close File(refnum=w345) -> (error out=w346:errorcluster)  [unwired: 1 in, 1 out]
          n140 = call <vilib>:"Simple Error Handler.vi"("error in (no error)"=w346) -> ()  [unwired: 4 in, 5 out]
        }
      }
      n141 = VISA Clear(VISA resource name=w330, error in (no error)=w329) -> (VISA resource name out=w328:refnum<visa-resource-name>, error out=w327:errorcluster)
      n142 = VISA Write(VISA resource name=w328, write buffer="pause stream (Teensy char)", error in (no error)=w327) -> (VISA resource name out=w339:refnum<visa-resource-name>, error out=w338:errorcluster)  [unwired: 1 out]
      n143 = VISA Read(VISA resource name=w339, byte count=u32 20000, error in (no error)=w338) -> (VISA resource name out=w335:refnum<visa-resource-name>, read buffer=→"Text response":string, error out=w333:errorcluster)  [unwired: 1 out]
      n144 = VISA Clear(VISA resource name=w335, error in (no error)=w333) -> (VISA resource name out=w334:refnum<visa-resource-name>, error out=w332:errorcluster)
      n145 = VISA Close(VISA resource name=w334, error in (no error)=w332) -> (error out=→"error out":errorcluster)
    }
  }
